vi "ini output cluster.vi"(0 "recipients":string[](array[string])=["nmswyers@gmail.com"] caption="Email Recipients", 1 "time stamp":timestamp, 2 "hours old date mod(hours)":u8=2, 3 "File Management":T2, 4 "Auto FTP":bool, 6 "Auto Archive":bool, 7 "Email Notification Cluster":T1, 9 "FTP Creds":T3={"Host"="", "UserName"="", "PassWord"="", "FTP File Path"="", "FTP Timeout (S)"=60, "Active or Passive"=FALSE, "ASCII or Binary"=FALSE} {"FTP Timeout (S)" min=0 max=300 step=1}, 11 "error in (no error)":errorcluster, 12 "File Path Cluster":T4={"Archive Location"=path "", "Archive Location 2"=path "<Not A Path>", "OutPut Path"=path "", "Directory(s) To Scan Files"=[]}, 14 "SITE ID":string="Site Not Configured" caption="Site ID:") -> (15 "error out":errorcluster)   [LabVIEW 2011]
uses:
  <vilib>/Utility/config.llb/NI_LVConfig.lvlib
  <vilib>/Utility/config.llb/Write Key (Path).vi
  <vilib>/Utility/config.llb/Write Key (String).vi
  <vilib>/Utility/config.llb/Write Key (I32).vi
  <vilib>/Utility/config.llb/Write Key (Boolean).vi
  <vilib>/Utility/config.llb/Write Key (U32).vi
  Controls/File Path directories.ctl
  Controls/FTP Credintials.ctl
  Controls/File Management.ctl
  Controls/Ping address and email notify.ctl
panel:
  # "File Handling Method"
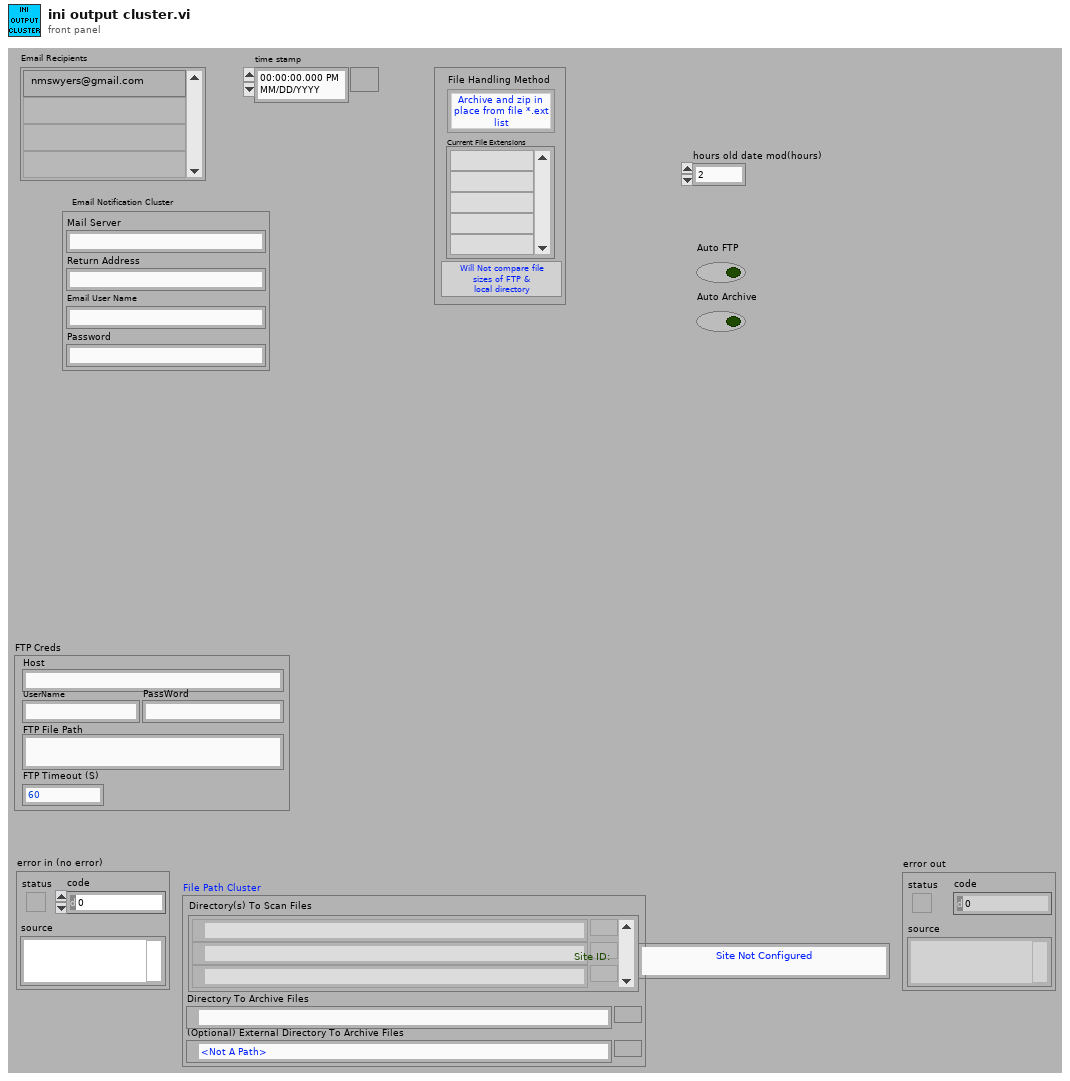
[diagram p1: front panel]
types:
  T1 = typedef "Ping address and email notify.ctl" = cluster{"Mail Server":string, "Return Address":string, "Email User Name":string, "Password":string}
  T2 = typedef "File Management.ctl" = cluster{"Comp File Size":bool, "File Handle Method":enum16{"Archive and zip in place from file *.ext list", "Archive and zip ALL file Types to archive directory", "Archive and zip to archive directory from file *.ext list", "Perform no file management"}, "file extention list":string[]}
  T3 = typedef "FTP Credintials.ctl" = cluster{"Host":string, "UserName":string, "PassWord":string, "FTP File Path":string, "FTP Timeout (S)":i32, "Active or Passive":bool, "ASCII or Binary":bool}
  T4 = typedef "File Path directories.ctl" = cluster{"Archive Location":path, "Archive Location 2":path, "OutPut Path":path, "Directory(s) To Scan Files":path[]}
  T5 = enum16{"Archive and zip in place from file *.ext list", "Archive and zip ALL file Types to archive directory", "Archive and zip to archive directory from file *.ext list", "Perform no file management"}
  T6 = typedef "NI_LVConfig.lvlib/Config Data RefNum.ctl" = refnum<k1>
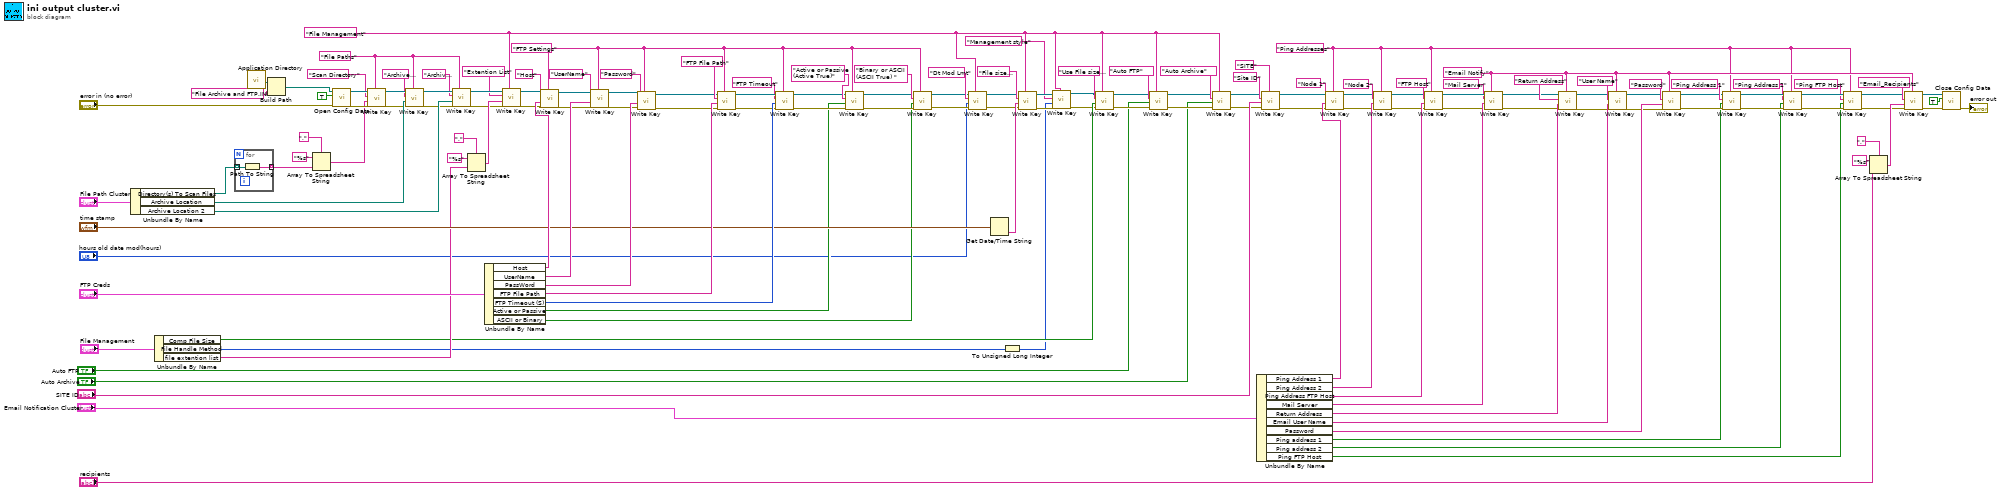
[diagram p0: block diagram]
diagram:
  w29 = "File Management" ("section")
  w7 = "Email Notify" ("name or relative path")
  w1 = "Ping Addresses" ("name or relative path")
  w44 = "FTP Settings" ("name or relative path")
  w92 = "File Paths" ("name or relative path")
  n1 = Unbundle By Name("File Path Cluster") -> ("Directory(s) To Scan Files"=w49:path[], "Archive Location"=w146:path, "Archive Location 2"=w147:path)
  n2 = Unbundle By Name("File Management") -> ("Comp File Size"=w57:bool, "File Handle Method"=w35:T5, "file extention list"=w58:string[])
  n3 = for {
    tunnel: w49 -> [w149] mode=indexing
    tunnel: [w148] -> w46 mode=indexing
    n4 = Path To String(path=w149) -> (string=w148:string)
  }
  n5 = call <vilib>:"Application Directory.vi"() -> ("Application Directory"=w20:path)
  n6 = Build Path(base path=w20, name or relative path="File Archive and FTP.INI") -> (appended path=w18:path)
  n7 = Array To Spreadsheet String(delimiter (Tab)=",", array=w46, 3:"%s" ("format string")) -> (spreadsheet string=w45:string)
  n8 = call <vilib>:"Open Config Data.vi"("error in (no error)"="error in (no error)", "create file if necessary (T)"=TRUE, "configuration file path"=w18) -> ("error out"=w99:errorcluster, "refnum"=w98:T6)  [unwired: 6 in, 1 out]
  n9 = call-poly <vilib>:"Write Key.vi"("section"=w92, "error in (no error)"=w99, "value"=w45, "key"="Scan Directory" ("name or relative path"), "refnum"=w98) -> ("error out"=w96:errorcluster, "refnum out"=w97:T6)  [unwired: 4 in, 1 out]
  n10 = call-poly <vilib>:"Write Key.vi"("section"=w92, "error in (no error)"=w96, "value"=w146, "key"="Archive location 1" ("name or relative path"), "refnum"=w97) -> ("error out"=w94:errorcluster, "refnum out"=w95:T6)  [unwired: 4 in, 1 out]
  n11 = call-poly <vilib>:"Write Key.vi"("section"=w92, "error in (no error)"=w94, "value"=w147, "key"="Archive location 2" ("name or relative path"), "refnum"=w95) -> ("error out"=w63:errorcluster, "refnum out"=w65:T6)  [unwired: 4 in, 1 out]
  n12 = Array To Spreadsheet String(delimiter (Tab)=",", array=w58, 3:"%s" ("format string")) -> (spreadsheet string=w66:string)
  n13 = Unbundle By Name("FTP Creds") -> ("Host"=w101:string, "UserName"=w102:string, "PassWord"=w103:string, "FTP File Path"=w104:string, "FTP Timeout (S)"=w105:i32, "Active or Passive"=w61:bool, "ASCII or Binary"=w60:bool)
  n14 = call-poly <vilib>:"Write Key.vi"("section"=w29, "error in (no error)"=w63, "value"=w66, "key"="Extention List", "refnum"=w65) -> ("error out"=w62:errorcluster, "refnum out"=w64:T6)  [unwired: 4 in, 1 out]
  n15 = call-poly <vilib>:"Write Key.vi"("section"=w44, "error in (no error)"=w62, "value"=w101, "key"="Host" ("name or relative path"), "refnum"=w64) -> ("error out"=w88:errorcluster, "refnum out"=w85:T6)  [unwired: 4 in, 1 out]
  n16 = call-poly <vilib>:"Write Key.vi"("section"=w44, "error in (no error)"=w88, "value"=w102, "key"="UserName" ("name or relative path"), "refnum"=w85) -> ("error out"=w87:errorcluster, "refnum out"=w84:T6)  [unwired: 4 in, 1 out]
  n17 = call-poly <vilib>:"Write Key.vi"("section"=w44, "error in (no error)"=w87, "value"=w103, "key"="Password" ("name or relative path"), "refnum"=w84) -> ("error out"=w43:errorcluster, "refnum out"=w42:T6)  [unwired: 4 in, 1 out]
  n18 = call-poly <vilib>:"Write Key.vi"("section"=w44, "error in (no error)"=w43, "value"=w104, "key"="FTP File Path" ("name or relative path"), "refnum"=w42) -> ("error out"=w86:errorcluster, "refnum out"=w83:T6)  [unwired: 4 in, 1 out]
  n19 = call-poly <vilib>:"Write Key.vi"("section"=w44, "error in (no error)"=w86, "value"=w105, "key"="FTP Timeout" ("name or relative path"), "refnum"=w83) -> ("error out"=w69:errorcluster, "refnum out"=w70:T6)  [unwired: 4 in, 1 out]
  n20 = call-poly <vilib>:"Write Key.vi"("section"=w44, "error in (no error)"=w69, "value"=w61, "key"="Active or Passive (Active True)" ("name or relative path"), "refnum"=w70) -> ("error out"=w135:errorcluster, "refnum out"=w136:T6)  [unwired: 4 in, 1 out]
  n21 = call-poly <vilib>:"Write Key.vi"("section"=w44, "error in (no error)"=w135, "value"=w60, "key"="Binary or ASCII (ASCII True) " ("name or relative path"), "refnum"=w136) -> ("error out"=w38:errorcluster, "refnum out"=w40:T6)  [unwired: 4 in, 1 out]
  n22 = call-poly <vilib>:"Write Key.vi"("section"=w29, "error in (no error)"=w38, "value"="hours old date mod(hours)", "key"="Dt Mod Lmt" ("name or relative path"), "refnum"=w40) -> ("error out"=w37:errorcluster, "refnum out"=w39:T6)  [unwired: 4 in, 1 out]
  n23 = Get Date/Time String(seconds (now)="time stamp") -> (time string=w72:string)  [unwired: 2 in, 1 out]
  n24 = To Unsigned Long Integer(number=w35) -> (unsigned 32bit integer=w34:u32)
  n25 = call-poly <vilib>:"Write Key.vi"("section"=w29, "error in (no error)"=w37, "value"=w72, "key"="File size Compare (FTP to DIR)" ("name or relative path"), "refnum"=w39) -> ("error out"=w54:errorcluster, "refnum out"=w53:T6)  [unwired: 4 in, 1 out]
  n26 = call-poly <vilib>:"Write Key.vi"("section"=w29, "error in (no error)"=w54, "value"=w34, "key"="Management style", "refnum"=w53) -> ("error out"=w51:errorcluster, "refnum out"=w52:T6)  [unwired: 4 in, 1 out]
  n27 = call-poly <vilib>:"Write Key.vi"("section"=w29, "error in (no error)"=w51, "value"=w57, "key"="Use File size Compare (FTP to DIR)" ("name or relative path"), "refnum"=w52) -> ("error out"=w27:errorcluster, "refnum out"=w28:T6)  [unwired: 4 in, 1 out]
  n28 = call-poly <vilib>:"Write Key.vi"("section"=w29, "error in (no error)"=w27, "value"="Auto FTP", "key"="Auto FTP" ("name or relative path"), "refnum"=w28) -> ("error out"=w25:errorcluster, "refnum out"=w26:T6)  [unwired: 4 in, 1 out]
  n29 = call-poly <vilib>:"Write Key.vi"("section"=w29, "error in (no error)"=w25, "value"="Auto Archive", "key"="Auto Archive" ("name or relative path"), "refnum"=w26) -> ("error out"=w21:errorcluster, "refnum out"=w22:T6)  [unwired: 4 in, 1 out]
  n30 = Unbundle By Name("Email Notification Cluster") -> ("Ping Address 1"=w139:string, "Ping Address 2"=w140:string, "Ping Address FTP Host"=w141:string, "Mail Server"=w142:string, "Return Address"=w143:string, "Email User Name"=w144:string, "Password"=w145:string, "Ping address 1"=w4:bool, "Ping address 2"=w3:bool, "Ping FTP Host"=w2:bool)
  n31 = call-poly <vilib>:"Write Key.vi"("section"="SITE" ("name or relative path"), "error in (no error)"=w21, "value"="SITE ID", "key"="Site ID" ("name or relative path"), "refnum"=w22) -> ("error out"=w116:errorcluster, "refnum out"=w115:T6)  [unwired: 4 in, 1 out]
  n32 = call-poly <vilib>:"Write Key.vi"("section"=w1, "error in (no error)"=w116, "value"=w139, "key"="Node 1" ("Mail Server"), "refnum"=w115) -> ("error out"=w117:errorcluster, "refnum out"=w111:T6)  [unwired: 4 in, 1 out]
  n33 = call-poly <vilib>:"Write Key.vi"("section"=w1, "error in (no error)"=w117, "value"=w140, "key"="Node 2" ("Mail Server"), "refnum"=w111) -> ("error out"=w118:errorcluster, "refnum out"=w110:T6)  [unwired: 4 in, 1 out]
  n34 = call-poly <vilib>:"Write Key.vi"("section"=w1, "error in (no error)"=w118, "value"=w141, "key"="FTP Host" ("Mail Server"), "refnum"=w110) -> ("error out"=w131:errorcluster, "refnum out"=w130:T6)  [unwired: 4 in, 1 out]
  n35 = call-poly <vilib>:"Write Key.vi"("section"=w7, "error in (no error)"=w131, "value"=w142, "key"="Mail Server" ("Mail Server"), "refnum"=w130) -> ("error out"=w125:errorcluster, "refnum out"=w124:T6)  [unwired: 4 in, 1 out]
  n36 = call-poly <vilib>:"Write Key.vi"("section"=w7, "error in (no error)"=w125, "value"=w143, "key"="Return Address" ("Return Address"), "refnum"=w124) -> ("error out"=w123:errorcluster, "refnum out"=w120:T6)  [unwired: 4 in, 1 out]
  n37 = call-poly <vilib>:"Write Key.vi"("section"=w7, "error in (no error)"=w123, "value"=w144, "key"="User Name" ("Email User Name"), "refnum"=w120) -> ("error out"=w122:errorcluster, "refnum out"=w121:T6)  [unwired: 4 in, 1 out]
  n38 = call-poly <vilib>:"Write Key.vi"("section"=w7, "error in (no error)"=w122, "value"=w145, "key"="Password" ("Password"), "refnum"=w121) -> ("error out"=w14:errorcluster, "refnum out"=w15:T6)  [unwired: 4 in, 1 out]
  n39 = call-poly <vilib>:"Write Key.vi"("section"=w1, "error in (no error)"=w14, "value"=w4, "key"="Ping Address 1" ("Password"), "refnum"=w15) -> ("error out"=w13:errorcluster, "refnum out"=w8:T6)  [unwired: 4 in, 1 out]
  n40 = call-poly <vilib>:"Write Key.vi"("section"=w1, "error in (no error)"=w13, "value"=w3, "key"="Ping Address 2" ("Password"), "refnum"=w8) -> ("error out"=w12:errorcluster, "refnum out"=w9:T6)  [unwired: 4 in, 1 out]
  n41 = call-poly <vilib>:"Write Key.vi"("section"=w1, "error in (no error)"=w12, "value"=w2, "key"="Ping FTP Host" ("Password"), "refnum"=w9) -> ("error out"=w11:errorcluster, "refnum out"=w10:T6)  [unwired: 4 in, 1 out]
  n42 = Array To Spreadsheet String(delimiter (Tab)=",", array="recipients", 3:"%s" ("format string")) -> (spreadsheet string=w134:string)
  n43 = call-poly <vilib>:"Write Key.vi"("section"=w7, "error in (no error)"=w11, "value"=w134, "key"="Email_Recipients" ("Password"), "refnum"=w10) -> ("error out"=w32:errorcluster, "refnum out"=w33:T6)  [unwired: 4 in, 1 out]
  n44 = call <vilib>:"Close Config Data.vi"("error in (no error)"=w32, "write file if changed (T)"=TRUE, "refnum"=w33) -> ("error out"=→"error out":errorcluster)  [unwired: 7 in, 1 out]
